vi "CMD_TRANSFORML2G.vi"(6 "Gantry in":refnum<class "Gantry.lvclass">, 8 "error in (no error)":errorcluster, 10 "Arguments":string[](array[string]), 11 "gScript Interpreter in":refnum<class "gScript Interpreter.lvclass">) -> (0 "error out":errorcluster, 3 "gScript Interpreter out":refnum<class "gScript Interpreter.lvclass">, 4 "Gantry out":refnum<class "Gantry.lvclass">)   [LabVIEW 2023, in "gScript Interpreter.lvclass"]
uses:
  gScript Interpreter.lvclass
  Shared Components/Gantry Class/Gantry.lvclass
  Shared Components/Utils/Type Definitions/Position_Orientation.ctl
  Shared Components/Vec3d Class/Vec3d.lvclass
  Shared Components/Orient3d Class/Orient3d.lvclass
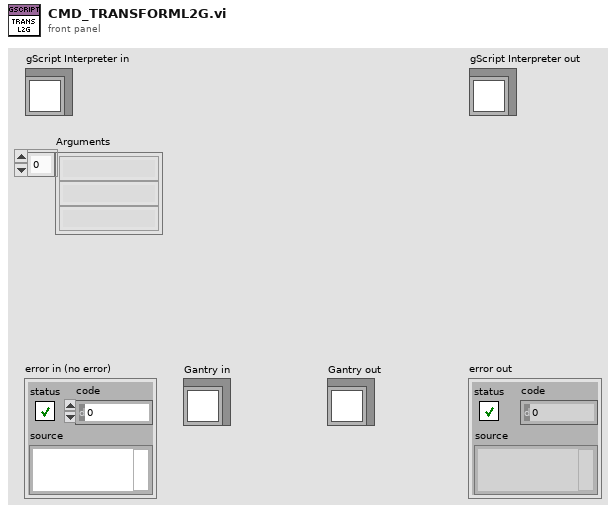
[diagram p1: front panel]
types:
  T1 = typedef "Position_Orientation.ctl" = cluster{"Center":refnum<class "Vec3d.lvclass">, "Orientation":refnum<class "Orient3d.lvclass">}
  T2 = typedef "Memory Cell.ctl" = cluster{"type":T3, "x":dbl, "y":dbl, "z":dbl, "w":dbl}
  T3 = typedef "Memory Cell Type Enum.ctl" = enum16{"integer", "float", "vector", "rotation"}
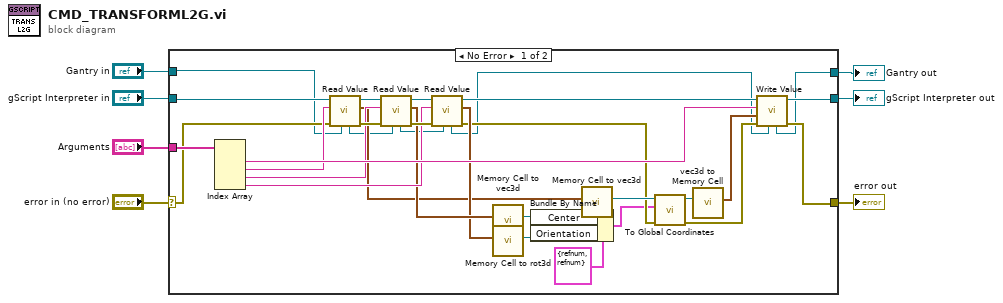
[diagram p0: block diagram]
diagram:
  n1 = case shown="No Error" "error in (no error)" {
    selector: "error in (no error)" -> [w20 w41]
    tunnel: [w19 w41] -> w6
    tunnel: [w18 w40] -> w4
    tunnel: "gScript Interpreter in" -> [w21 w40]
    tunnel: "Arguments" -> [w22 _]
    tunnel: "Gantry in" -> [w12 w39]
    tunnel: [w8 w39] -> w1
    frame No Error {
      n2 = Index Array(array=w22) -> (element #1=w38:string, element #2=w37:string, element #3=w32:string, element #4=w31:string)  [unwired: 4 in]
      n3 = call-dynamic "Read Value.vi"("Gantry in"=w12, "error in (no error)"=w20, "String in"=w37, "gScript Interpreter in"=w21) -> ("error out"=w34:errorcluster, "Memory Cell"=w25:T2, "gScript Interpreter out"=w36:refnum<class "gScript Interpreter.lvclass">, "Gantry out"=w11:refnum<class "Gantry.lvclass">)  [unwired: 4 in]
      n4 = call-dynamic "Read Value.vi"("Gantry in"=w11, "error in (no error)"=w34, "String in"=w32, "gScript Interpreter in"=w36) -> ("error out"=w33:errorcluster, "Memory Cell"=w27:T2, "gScript Interpreter out"=w35:refnum<class "gScript Interpreter.lvclass">, "Gantry out"=w10:refnum<class "Gantry.lvclass">)  [unwired: 4 in]
      n5 = call-dynamic "Read Value.vi"("Gantry in"=w10, "error in (no error)"=w33, "String in"=w31, "gScript Interpreter in"=w35) -> ("error out"=w15:errorcluster, "Memory Cell"=w26:T2, "gScript Interpreter out"=w24:refnum<class "gScript Interpreter.lvclass">, "Gantry out"=w9:refnum<class "Gantry.lvclass">)  [unwired: 4 in]
      n6 = call "Memory Cell to vec3d.vi"("Memory Cell"=w27) -> ("Vec3d out"=w29:refnum<class "Vec3d.lvclass">)  [unwired: 10 in]
      n7 = call "Memory Cell to rot3d.vi"("Memory Cell"=w26) -> ("Orient3d out"=w28:refnum<class "Orient3d.lvclass">)  [unwired: 10 in]
      n8 = Bundle By Name(cluster=T1 {"Center"=refnum, "Orientation"=refnum} ("Center/Orientation"), "Center"=w29, "Orientation"=w28) -> (w14:T1)
      n9 = call "Memory Cell to vec3d.vi"("Memory Cell"=w25) -> ("Vec3d out"=w17:refnum<class "Vec3d.lvclass">)  [unwired: 10 in]
      n10 = call "To Global Coordinates.vi"("error in"=w15, "Center/Orientation"=w14, "Local Coordinates"=w17) -> ("error out"=w16:errorcluster, "Global Coordinates"=w13:refnum<class "Vec3d.lvclass">)  [unwired: 7 in]
      n11 = call "vec3d to Memory Cell.vi"("Vec3d in"=w13) -> ("Memory Cell"=w23:T2)  [unwired: 10 in]
      n12 = call-dynamic "Write Value.vi"("Gantry in"=w9, "error in (no error)"=w16, "Value"=w23, "Address"=w38, "gScript Interpreter in"=w24) -> ("error out"=w19:errorcluster, "gScript Interpreter out"=w18:refnum<class "gScript Interpreter.lvclass">, "Gantry out"=w8:refnum<class "Gantry.lvclass">)  [unwired: 4 in]
    }
    frame Error {
    }
  }
  "error out" <- w6
  "gScript Interpreter out" <- w4
  "Gantry out" <- w1
